vi "输出调用04.vi"(0 "输出簇":cluster{"用户名":string, "项目名称":string}, 7 "数组":string[][](array[string]), 9 "字符串":string, 11 "输出簇 2":T1) -> ()   [LabVIEW 2020]
uses:
  <vilib>/Utility/miscctls.llb/LVDateTimeRec.ctl
panel:
  out "数组 6":dbl[][](array[numeric])
  out "水质":dbl
  out "温度":dbl
  out "输出 3":dbl
  out "输出 2":dbl
  out "创建的路径":path
  out "路径 2":path
  out "路径":path
  out "错误输出":errorcluster
  out "数组 5":dbl[](array[numeric])
  out "数组 4":dbl[](array[numeric])
  out "文本":string[](array[string])
  out "数组 3":dbl[](array[numeric])
  out "数组 2":dbl[](array[numeric])
  out "错误输出 2":errorcluster caption="错误输出"
  out "元素":string
  out "数值 3":i32
  out "Numeric":i32
  in  "数值":u32
  out "输出 1":dbl
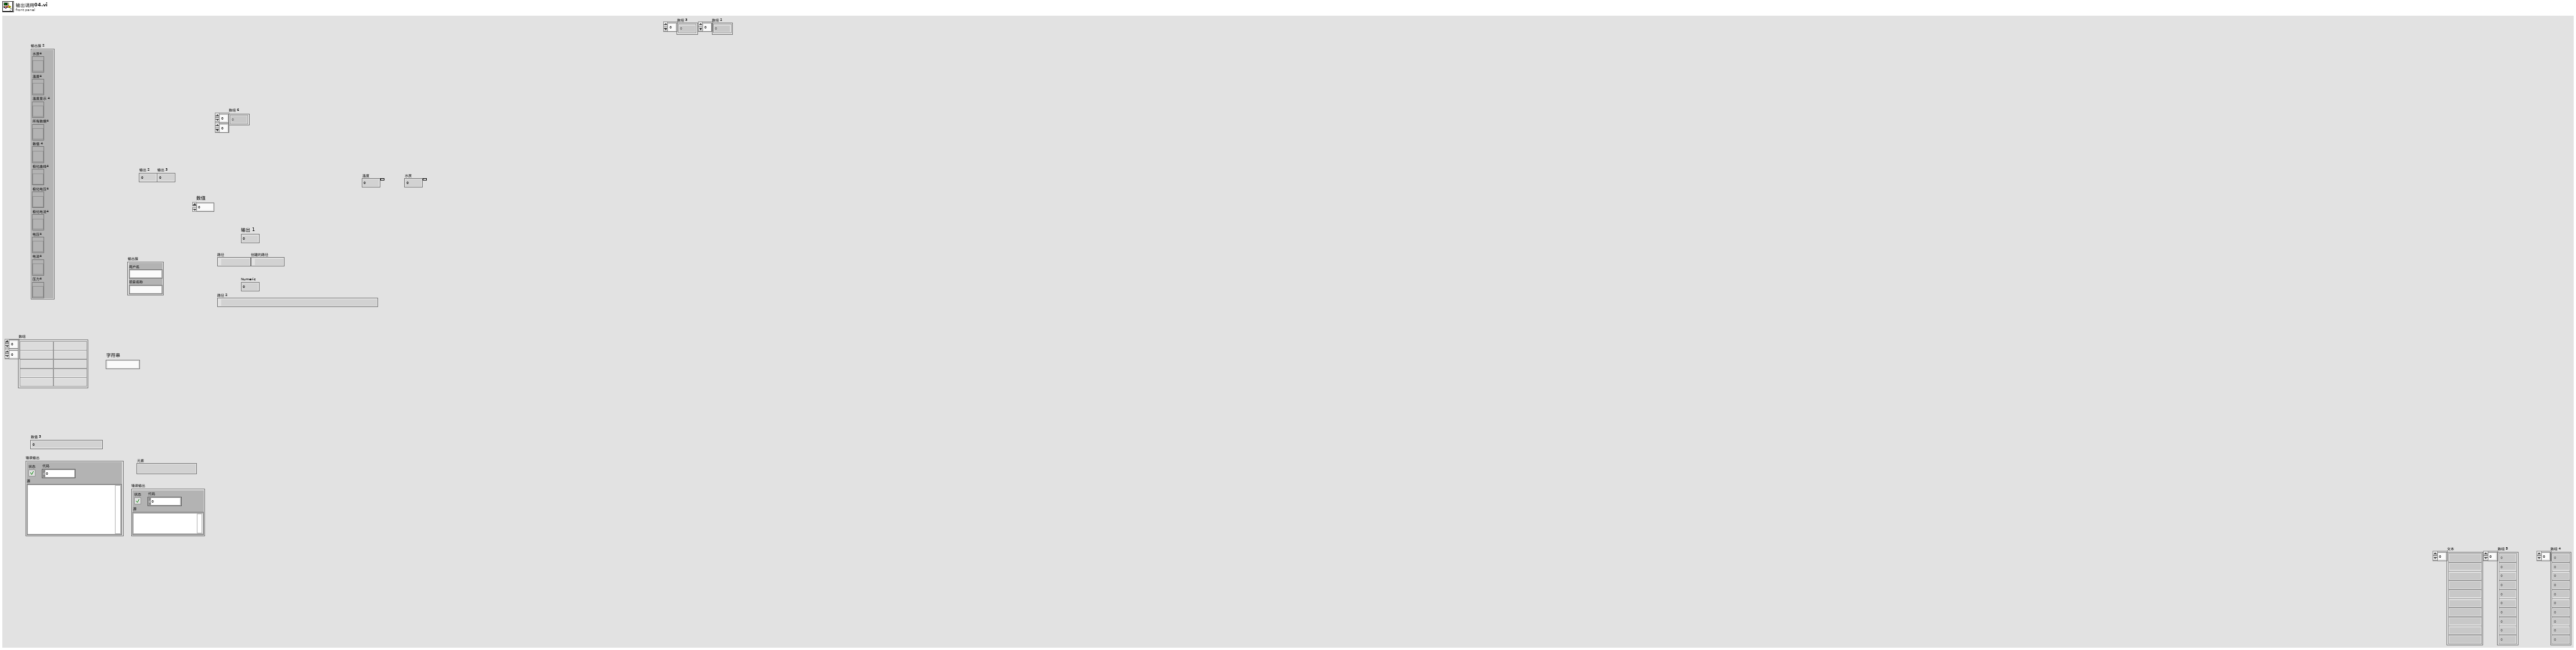
[diagram p1: front panel]
types:
  T1 = cluster{"水质4":refnum<vi>, "温度4":refnum<vi>, "温度显示 4":refnum<vi>, "所有数据4":refnum<vi>, "数值 4":refnum<vi>, "极化曲线4":refnum<vi>, "极化电压4":refnum<vi>, "极化电流4":refnum<vi>, "电压4":refnum<vi>, "电流4":refnum<vi>, "压力4":refnum<vi>}
  T2 = enum16{"open", "replace", "create", "open or create", "replace or create", "replace or create with confirmation"}
  T3 = typedef "LVDateTimeRec.ctl" = cluster{"fractional second":dbl, "second":i32, "minute":i32, "hour":i32, "day of month":i32, "month":i32, "year":i32, "day of week":i32, "day of year":i32, "DST":i32}
  T4 = enum16{"open", "open or create", "create or replace", "create", "open (read-only)"}
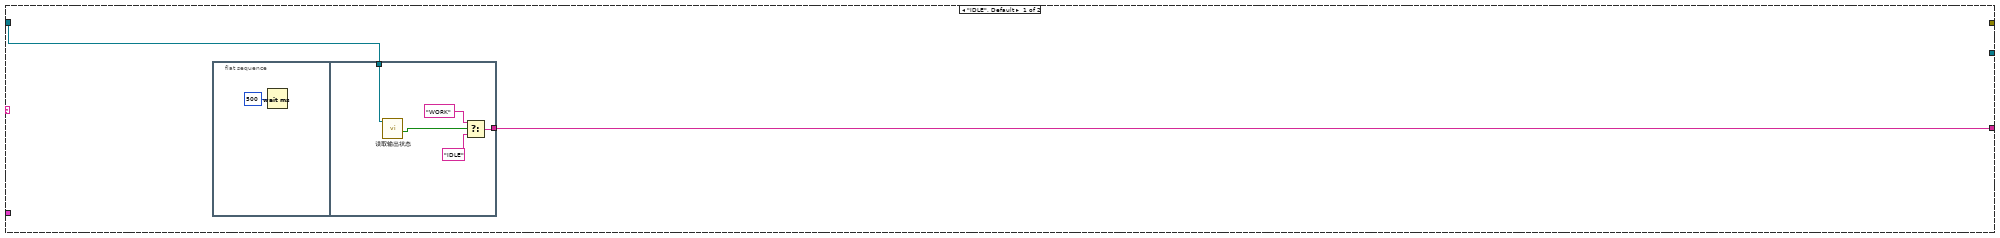
[diagram p2: hidden frame]
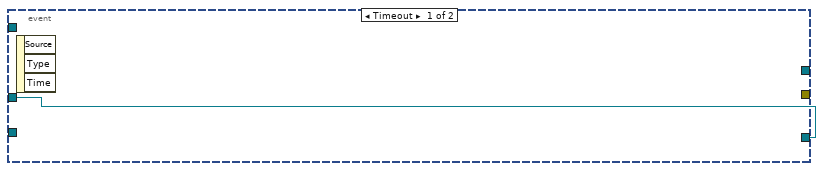
[diagram p3: hidden frame]
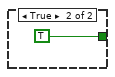
[diagram p5: hidden frame]
diagram:
  w12 = "\\" ("string")
  (unwired) dbl[] [] ("数组 4")
  n1 = Current VI's Path() -> (path=w36:path)
  n2 = Strip Path(path=w36) -> (stripped path=w35:path)  [unwired: 1 out]
  n3 = Strip Path(path=w35) -> (stripped path=w34:path)  [unwired: 1 out]
  n4 = Path To String(path=w34) -> (string=w33:string)
  n5 = Unbundle By Name("输出簇") -> ("用户名"=w9:string, "项目名称"=w8:string)
  n6 = Get Date/Time In Seconds() -> (seconds since 1Jan1904=w31:timestamp)
  n7 = Format Date/Time String(time format string (%c)="%y-%m-%d[%H-%M]", seconds (now)=w31) -> (date/time string=w11:string)  [unwired: 1 in]
  n8 = Concatenate Strings(w33, w12, "TEMPDATA\\" ("string"), w9, w12, w8, w12, w11) -> (w29:string)
  n9 = String To Path(string=w29) -> (path=w28:path)
  n10 = Create Folder(path (use dialog)=w28) -> (created path=w21:path)  [unwired: 2 in, 2 out]
  "创建的路径" <- w21
  n11 = Path To String(path=w21) -> (string=w27:string)
  n12 = Concatenate Strings(w27, "\\" ("string"), "索引.txt" ("string")) -> (w18:string)
  n13 = String To Path(string=w18) -> (path=w17:path)
  "路径 2" <- w17
  n14 = property on="输出簇 2" class="Clust (严格)"() -> ("Value"=w1:T1)  [unwired: 2 in, 2 out]
  n15 = Unbundle By Name(w1) -> ("极化曲线4"=w7:refnum<vi>)
  n16 = property on="数组 6" class="Arr (严格)"("Value"=dbl[][] [] ("数组 6")) -> (error out=w3:errorcluster)  [unwired: 2 in, 1 out]
  n17 = Open/Create/Replace File(file path (use dialog)=w17, operation (0:open)=T2."replace or create") -> (refnum out=w16:refnum<file>)  [unwired: 4 in, 2 out]
  n18 = while {
    tunnel: w45 -> [w66]
    tunnel: w16 -> [w65]
    tunnel: [w64] -> w14
    tunnel: [w63] -> w15
    shift-right: [w61] -> _
    shift-left: w7 -> [w62]
    tunnel: w3 -> [_]
    stop <- FALSE stop-if-true
    n19 = event shown="[1] \"数值\": 值改变" {
      selector: _ -> [_ _]
      dyn-events: _ -> [_ _]
      timeout: 100 -> [_ _]
      tunnel: w66 -> [_ _]
      tunnel: w65 -> [_ w84]
      tunnel: [_ w78] -> w64
      tunnel: [_ w77] -> w63
      tunnel: w62 -> [w69 w73]
      tunnel: [w69 w72] -> w61
      event Timeout {
        n20 = event-data() -> ()  [unwired: 1 in, 3 out]
      }
      event "数值": Value Change {
        n21 = event-data() -> ()  [unwired: 1 in, 6 out]
        n22 = local read "输出 3"() -> (w74:dbl)
        n23 = local read "输出 2"() -> (w75:dbl)
        n24 = property on="Numeric" class="DigNum (严格)"() -> ("Value"=w83:i32)  [unwired: 2 in, 2 out]
        n25 = Build Array(w75, w74) -> (w76:dbl[])
        n26 = Format Into String(w83) -> (resulting string=w82:string)  [unwired: 3 in, 1 out]
        n27 = property on="数组 6" class="Arr (严格)"() -> ("Value"=w71:dbl[][])  [unwired: 2 in, 2 out]
        n28 = Write to Text File(file (use dialog)=w84, text=w82) -> (refnum out=w81:refnum<file>, error out=w80:errorcluster)  [unwired: 2 in, 1 out]
        n29 = Insert Into Array(array=w71, new element=w76) -> (w70:dbl[][])  [unwired: 2 in]
        n30 = property on="数组 6" class="Arr (严格)"("Value"=w70) -> ()  [unwired: 2 in, 2 out]
        n31 = Write to Text File(file (use dialog)=w81, text="\r\n", error in=w80) -> (refnum out=w78:refnum<file>, error out=w77:errorcluster)  [unwired: 1 in, 1 out]
        n32 = property class="Arr (严格)"(reference=w73, "Value"=w70) -> (reference out=w72:refnum<vi>)  [unwired: 1 in, 1 out]
      }
    }
  }
  n33 = Close File(refnum=w14, error in=w15) -> ()  [unwired: 2 out]
  n34 = Path To String(path=w21) -> (string=w22:string)
  n35 = Concatenate Strings(w22, "\\" ("string"), "数据.txt" ("string")) -> (w20:string)
  n36 = String To Path(string=w20) -> (path=w19:path)
  "路径" <- w19
  n37 = Open/Create/Replace File(file path (use dialog)=w19, operation (0:open)=T2."replace or create" ("操作(0:open)")) -> (refnum out=w5:refnum<file>, error out=w40:errorcluster)  [unwired: 4 in, 1 out]
  n38 = flat-sequence {
    tunnel: [w89] -> w60
    tunnel: [w86] -> w57
    tunnel: w60 -> [w93]
    tunnel: [w93] -> w59
    tunnel: [w92] -> w58
    tunnel: w57 -> [w92]
    tunnel: ["字符串"] -> w43
    tunnel: w59 -> [w95]
    tunnel: w58 -> [w96]
    tunnel: [w96] -> w56
    tunnel: [w95] -> w55
    tunnel: [w94] -> w44
    tunnel: w43 -> [w94]
    tunnel: w56 -> [w103]
    tunnel: w55 -> [w104]
    tunnel: [w106] -> w54
    tunnel: [w105] -> w53
    tunnel: [w104] -> w51
    tunnel: [w103] -> w49
    tunnel: [w102] -> w45
    tunnel: w44 -> [w101]
    tunnel: w54 -> [w119]
    tunnel: w53 -> [w118]
    tunnel: [w115] -> w52
    tunnel: w51 -> [w115]
    tunnel: [w114] -> w50
    tunnel: w49 -> [w114]
    tunnel: [w109] -> w48
    tunnel: [w108] -> w47
    tunnel: ["输出簇 2"] -> w6
    tunnel: w52 -> [w148]
    tunnel: w50 -> [w152]
    tunnel: w48 -> [w151]
    tunnel: w47 -> [w150]
    tunnel: [w149] -> w46
    tunnel: [w145] -> w37
    tunnel: w6 -> [w144]
    tunnel: w46 -> [w205]
    tunnel: w37 -> [w203]
    frame #0 {
      n39 = property on="数值" class="DigNum (严格)"("Value"=i64 0 ("数值")) -> ()  [unwired: 2 in, 2 out]
      n40 = Index Array(array="数组", index (col)=5 ("禁用的索引 (列)")) -> (element=w86:string[])  [unwired: 1 in]
      n41 = Index Array(array="数组", index (col)=3 ("禁用的索引 (列)")) -> (element=w89:string[])  [unwired: 1 in]
    }
    frame #1 {
      n42 = VISA Close(VISA resource name="字符串") -> ()  [unwired: 1 in, 1 out]
    }
    frame #2 {
    }
    frame #3 {
      n43 = VISA Open(VISA resource name=w101) -> (VISA resource name=w102:refnum<visa-resource-name>, error out=w99:errorcluster)  [unwired: 4 in]
      n44 = call "remote.vi"("error in (no error)"=w99, "VISA resource name"=w102) -> ("error out"=w97:errorcluster, "VISA resource name out"=w98:refnum<visa-resource-name>)  [unwired: 8 in]
      n45 = call "enableoutput.vi"("error in (no error)"=w97, "Enable OutPut(True)"=FALSE, "VISA resource name"=w98) -> ("error out"=w105:errorcluster, "VISA resource name out"=w106:refnum<visa-resource-name>)  [unwired: 7 in]
    }
    frame #4 {
      n46 = flat-sequence {
        tunnel: w119 -> [w124]
        tunnel: w118 -> [w123]
        tunnel: [w121] -> w117
        tunnel: [w120] -> w116
        tunnel: w117 -> [w130]
        tunnel: w116 -> [w129]
        tunnel: [w126] -> w113
        tunnel: [w125] -> w112
        tunnel: w113 -> [w136]
        tunnel: w112 -> [w135]
        tunnel: [w133] -> w111
        tunnel: [w132] -> w110
        tunnel: w111 -> [w142]
        tunnel: w110 -> [w141]
        tunnel: [w138] -> w109
        tunnel: [w137] -> w108
        frame #0 {
          n47 = call "priority.vi"("error in (no error)"=w123, "字符串"="CURR", "VISA resource name"=w124) -> ("error out"=w120:errorcluster, "VISA resource name out"=w121:refnum<visa-resource-name>)  [unwired: 7 in]
        }
        frame #1 {
          n48 = call "初始化电压电流.vi"("error in (no error)"=w129, "输入 2"=0.1, "输入 1"=15.0, "VISA resource name"=w130) -> ("error out"=w125:errorcluster, "VISA resource name out"=w126:refnum<visa-resource-name>)  [unwired: 6 in]
        }
        frame #2 {
          n49 = call "限制电流.vi"("error in (no error)"=w135, "OCP Delay(0)"=3.0, "数值"=120.0 ("OCP Level(0)"), "VISA resource name"=w136) -> ("error out"=w132:errorcluster, "VISA resource name out"=w133:refnum<visa-resource-name>)  [unwired: 6 in]
        }
        frame #3 {
          n50 = call "限制电压.vi"("error in (no error)"=w141, "OVP Delay(0)"=3.0, "OVP Level(0)"=20.0, "VISA resource name"=w142) -> ("error out"=w137:errorcluster, "VISA resource name out"=w138:refnum<visa-resource-name>)  [unwired: 6 in]
        }
      }
    }
    frame #5 {
      n51 = Unbundle By Name(w144) -> ("数值 4"=w143:refnum<vi>)
      n52 = Search 1D Array(1D array=w148, element=" " ("元素")) -> (index of element=w146:i32)  [unwired: 1 in]
      n53 = for {
        N: w146 -> [_]
        tunnel: w152 -> [w174] mode=indexing
        tunnel: w148 -> [w171] mode=indexing
        tunnel: w150 -> [w169]
        shift-right: [w164] -> w149
        shift-left: w151 -> [w170]
        tunnel: [w161] -> w145
        shift-right: [w155] -> _
        shift-left: w143 -> [w156]
        i -> [w154]
        n54 = Scan From String(input string=w174) -> (output 1=w173:dbl)  [unwired: 4 in, 3 out]
        n55 = Scan From String(input string=w171) -> (output 1=w168:dbl)  [unwired: 4 in, 3 out]
        "输出 1" <- w168
        n56 = Multiply(x=w173, y=1000.0) -> (x*y=w165:dbl)
        n57 = flat-sequence {
          tunnel: w170 -> [w179]
          tunnel: w169 -> [w178]
          tunnel: w168 -> [w177]
          tunnel: [w176] -> w167
          tunnel: [w175] -> w166
          tunnel: w167 -> [w182]
          tunnel: w166 -> [w183]
          tunnel: [w181] -> w163
          tunnel: [w180] -> w162
          tunnel: w165 -> [w193]
          tunnel: w163 -> [w192]
          tunnel: [w192] -> w160
          tunnel: [w191] -> w158
          tunnel: w162 -> [w191]
          tunnel: w160 -> [w198]
          tunnel: [w198] -> w159
          tunnel: w158 -> [w197]
          tunnel: [w197] -> w157
          tunnel: w156 -> [w196]
          tunnel: [w195] -> w155
          tunnel: w153 -> [w194]
          tunnel: [w201] -> w164
          tunnel: w159 -> [w202]
          tunnel: w157 -> [w200]
          tunnel: [w199] -> w161
          frame #0 {
            n58 = call "设置电流.vi"("error in (no error)"=w178, "输入 1"=w177, "VISA resource name"=w179) -> ("error out"=w175:errorcluster, "VISA resource name out"=w176:refnum<visa-resource-name>)  [unwired: 7 in]
          }
          frame #1 {
            n59 = First Call?() -> (First Call?: T/F=w184:bool)
            n60 = case shown="真" w184 {
              tunnel: w182 -> [w185 w190]
              tunnel: w183 -> [_ w189]
              tunnel: [w185 w187] -> w181
              tunnel: [_ w186] -> w180
              frame False {
              }
              frame True {
                n61 = call "enableoutput.vi"("error in (no error)"=w189, "Enable OutPut(True)"=TRUE, "VISA resource name"=w190) -> ("error out"=w186:errorcluster, "VISA resource name out"=w187:refnum<visa-resource-name>)  [unwired: 7 in]
              }
            }
          }
          frame #2 {
            n62 = Wait (ms)(milliseconds to wait=w193) -> ()  [unwired: 1 out]
          }
          frame #3 {
            n63 = property on="数值" class="DigNum (严格)"("Val(Sgnl)"=w194) -> ()  [unwired: 2 in, 2 out]
            n64 = property class="DigNum (严格)"(reference=w196, "Val(Sgnl)"=w194) -> (reference out=w195:refnum<vi>)  [unwired: 1 in, 1 out]
          }
          frame #4 {
            n65 = call "remote.vi"("error in (no error)"=w200, "VISA resource name"=w202) -> ("error out"=w199:errorcluster, "VISA resource name out"=w201:refnum<visa-resource-name>)  [unwired: 8 in]
          }
        }
        n66 = Increment(x=w154) -> (x+1=w153:i32)
      }
    }
    frame #6 {
      n67 = flat-sequence {
        tunnel: w205 -> [w209]
        tunnel: [w208] -> w204
        tunnel: w203 -> [w206]
        tunnel: w204 -> [w210]
        frame #0 {
          n68 = call "enableoutput.vi"("error in (no error)"=w206, "Enable OutPut(True)"=FALSE, "VISA resource name"=w209) -> ("VISA resource name out"=w208:refnum<visa-resource-name>)  [unwired: 7 in, 1 out]
        }
        frame #1 {
          n69 = VISA Close(VISA resource name=w210) -> ()  [unwired: 1 in, 1 out]
        }
        frame #2 {
          n70 = flat-sequence {
            tunnel: [w227] -> w221
            tunnel: [w226] -> w220
            tunnel: [w225] -> w219
            tunnel: [w224] -> w218
            tunnel: [w223] -> w217
            tunnel: w221 -> [w270]
            tunnel: w220 -> [w269]
            tunnel: [w287] -> w211
            tunnel: [w286] -> w212
            tunnel: w219 -> [w282]
            tunnel: [w281] -> w213
            tunnel: w218 -> [w273]
            tunnel: w217 -> [w274]
            tunnel: [w271] -> w214
            tunnel: [w272] -> w215
            tunnel: [w271] -> w216
            tunnel: w216 -> [w328]
            tunnel: w215 -> [w327]
            tunnel: w214 -> [w349]
            tunnel: w213 -> [w355]
            tunnel: w212 -> [w363]
            tunnel: w211 -> [w362]
            frame #0 {
              n71 = property on="路径" class="Path"() -> ("Value"=w222:path)  [unwired: 2 in, 2 out]
              n72 = Open/Create/Replace File(file path (use dialog)=w222, operation (0:open)=T2."open" ("操作(0:open)")) -> (refnum out=w230:refnum<file>, error out=w229:errorcluster)  [unwired: 4 in, 1 out]
              n73 = while {
                tunnel: w230 -> [w266]
                tunnel: w229 -> [w264]
                tunnel: [w263] -> w228
                tunnel: [w237] -> w227 mode=indexing
                tunnel: [w236] -> w226 mode=indexing
                tunnel: [w252] -> _
                tunnel: [w240] -> w225 mode=indexing
                tunnel: [w235] -> w224 mode=indexing
                tunnel: [w234] -> w223 mode=indexing
                i -> [w233]
                stop <- w253 stop-if-true
                n74 = Read from Text File(file (use dialog)=w266, count=1 ("计数"), error in=w264) -> (refnum out=w263:refnum<file>, text=w257:string[], error out=w252:errorcluster)  [unwired: 1 in, 1 out]
                n75 = Unbundle By Name(w252) -> ("status"=w260:bool, "code"=w262:i32)
                n76 = Equal?(x=w262, y=4) -> (x = y?=w259:bool)
                n77 = Index Array(array=w257, index=0 ("索引")) -> (element=w254:string)
                "元素" <- w254
                n78 = And(x=w260, y=w259) -> (x .and. y?=w258:bool)
                n79 = case shown="假" w258 {
                  tunnel: [FALSE TRUE] -> w253
                  frame False {
                  }
                  frame True {
                  }
                }
                n80 = Search/Split String(string=w254, search string/char (-)="电流：" ("正则表达式")) -> (substring before match=w249:string, match + rest of string=w239:string)  [unwired: 1 in, 1 out]
                n81 = Scan From String(format string="%d-%d-%d %d:%d:%d" ("格式字符串"), input string=w249) -> (error out=→"错误输出 2":errorcluster, output 1=w248:i32, output 2=w247:i32, output 3=w246:i32, output 4=w245:i32, output 5=w244:i32, output 6=w243:i32)  [unwired: 8 in, 2 out]
                n82 = Bundle By Name(cluster=T3 {"fractional second"=0.9035696983337402, "second"=34, "minute"=35, "hour"=15, "day of month"=21, "month"=2, "year"=2022, "day of week"=2, "day of year"=52, "DST"=0} ("日期时间记录"), "second"=w243, "minute"=w244, "hour"=w245, "day of month"=w246, "month"=w247, "year"=w248) -> (w241:T3)
                n83 = Scan From String(format string="电流：%f 电压：%f 温度：%f 水质：%f" ("格式字符串"), input string=w239) -> (error out=w232:errorcluster, output 1=w237:dbl, output 2=w236:dbl, output 3=w235:dbl, output 4=w234:dbl)  [unwired: 6 in, 2 out]
                n84 = call <vilib>:"Clear Errors.vi"("error in (no error)"=w232) -> ()  [unwired: 5 in, 2 out]
                n85 = Date/Time To Seconds(2:w241) -> (0:w240:timestamp)  [unwired: 1 in]
                "数值 3" <- w233
              }
              n86 = Close File(refnum=w228) -> ()  [unwired: 1 in, 2 out]
            }
            frame #1 {
              n87 = Array Size(array=w269) -> (size(s)=w289:i32)
              n88 = Array Size(array=w270) -> (size(s)=w292:i32)
              n89 = Array Size(array=w282) -> (size(s)=w284:i32)
              n90 = Decrement(x=w289) -> (x-1=w290:i32)
              n91 = Decrement(x=w292) -> (x-1=w291:i32)
              n92 = Decrement(x=w284) -> (x-1=w285:i32)
              n93 = Array Size(array=w273) -> (size(s)=w280:i32)
              n94 = Array Size(array=w274) -> (size(s)=w279:i32)
              n95 = Decrement(x=w280) -> (x-1=w278:i32)
              n96 = Decrement(x=w279) -> (x-1=w275:i32)
              n97 = Delete From Array(array=w273, length=1 ("长度"), index=w278) -> (array with subset deleted=w271:dbl[])  [unwired: 1 out]
              n98 = Delete From Array(array=w269, length=1 ("长度"), index=w290) -> (array with subset deleted=w286:dbl[])  [unwired: 1 out]
              n99 = Delete From Array(array=w270, length=1 ("长度"), index=w291) -> (array with subset deleted=w287:dbl[])  [unwired: 1 out]
              n100 = Delete From Array(array=w282, length=1 ("长度"), index=w285) -> (array with subset deleted=w281:timestamp[])  [unwired: 1 out]
              n101 = Delete From Array(array=w274, length=1 ("长度"), index=w275) -> (array with subset deleted=w272:dbl[])  [unwired: 1 out]
              "数组 3" <- w270
              "数组 2" <- w269
            }
            frame #2 {
              w314 = "极化" ("组名称输入（无标题）")
              w340 = "数据" ("组名称")
              n102 = property on="创建的路径" class="Path"() -> ("Value"=w294:path)  [unwired: 2 in, 2 out]
              n103 = Array Max & Min(array=w349) -> (max value=w321:dbl, max index (indices)=w319:i32, min value=w320:dbl, min index (indices)=w318:i32)
              n104 = Array Max & Min(array=w327) -> (max value=w325:dbl, max index (indices)=w323:i32, min value=w324:dbl, min index (indices)=w322:i32)
              n105 = Array Size(array=w355) -> (size(s)=w354:i32)
              n106 = Array Max & Min(array=w363) -> (max value=w376:dbl, max index (indices)=w371:i32, min value=w375:dbl, min index (indices)=w370:i32)
              n107 = Array Max & Min(array=w362) -> (max value=w378:dbl, max index (indices)=w372:i32, min value=w379:dbl, min index (indices)=w373:i32)
              n108 = Index Array(array=w355, index=0 ("索引")) -> (element=w352:timestamp)
              n109 = Build Array(w325, w324, w323, w322) -> (w336:dbl[])
              n110 = Build Array(w321, w320, w319, w318) -> (w337:dbl[])
              n111 = Decrement(x=w354) -> (x-1=w353:i32)
              n112 = Build Array(w375, w376, w371, w370) -> (w374:dbl[])
              n113 = Build Array(w379, w378, w373, w372) -> (w377:dbl[])
              n114 = Path To String(path=w294) -> (string=w295:string)
              n115 = Index Array(array=w355, index=w353) -> (element=w351:timestamp)
              n116 = Get Date/Time In Seconds() -> (seconds since 1Jan1904=w395:timestamp)
              n117 = Format Date/Time String(time format string (%c)="%Y-%m-%d-%H-%M-%S" ("时间格式字符串(%c)"), seconds (now)=w395) -> (date/time string=w297:string)  [unwired: 1 in]
              n118 = Concatenate Strings(w295, "\\" ("字符串"), w297, ".tdms" ("字符串")) -> (w396:string)
              n119 = String To Path(string=w396) -> (path=w397:path)
              n120 = Build Array(w352, w351) -> (w350:timestamp[])
              n121 = TDMS Open(5:FALSE ("创建索引文件？(T)"), 10:T4."create or replace" ("操作(0:open)"), 11:w397) -> (0:w303:errorcluster, 3:w305:refnum<k34>)  [unwired: 4 in]
              n122 = Build Array("电解水实验" ("组名称"), "孙成，王彪" ("组名称"), w297, "极化曲线" ("组名称")) -> (w296:string[])
              n123 = TDMS Set Properties(5:w296, 7:string[] ["Title", "Author", "Date/Time", "type"] ("属性名称"), 8:w303, 11:w305) -> (0:w302:errorcluster, 3:w304:refnum<k34>)  [unwired: 2 in, 2 out]
              n124 = TDMS Set Properties(5:w350, 7:string[] ["最小值", "最大值"] ("属性名称"), 8:w302, 9:"测试时间" ("通道名称"), 10:w340, 11:w304) -> (0:w386:errorcluster, 3:w387:refnum<k34>)  [unwired: 2 out]
              n125 = TDMS Set Properties(5:w377, 7:string[] ["最小值", "最大值", "最小索引", "最大索引"] ("属性名称"), 8:w386, 9:"电流" ("通道名称"), 10:w340, 11:w387) -> (0:w380:errorcluster, 3:w383:refnum<k34>)  [unwired: 2 out]
              n126 = TDMS Set Properties(5:w374, 7:string[] ["最小值", "最大值", "最小索引", "最大索引"] ("属性名称"), 8:w380, 9:"电压" ("通道名称"), 10:w340, 11:w383) -> (0:w343:errorcluster, 3:w344:refnum<k34>)  [unwired: 2 out]
              n127 = TDMS Set Properties(5:w337, 7:string[] ["最小值", "最大值", "最小索引", "最大索引"] ("属性名称"), 8:w343, 9:"温度" ("通道名称"), 10:w340, 11:w344) -> (0:w341:errorcluster, 3:w342:refnum<k34>)  [unwired: 2 out]
              n128 = TDMS Set Properties(5:w336, 7:string[] ["最小值", "最大值", "最小索引", "最大索引"] ("属性名称"), 8:w341, 9:"水质" ("通道名称"), 10:w340, 11:w342) -> (0:w338:errorcluster, 3:w339:refnum<k34>)  [unwired: 2 out]
              n129 = TDMS Write(0:w339, 5:"数据" ("组名称输入（无标题）"), 7:string[] ["电流"] ("通道名输入（无标题）"), 9:w362, 11:w338) -> (4:w366:refnum<k34>, 15:w365:errorcluster)  [unwired: 1 in, 2 out]
              n130 = TDMS Write(0:w366, 5:"数据" ("组名称输入（无标题）"), 7:string[] ["电压"] ("通道名输入（无标题）"), 9:w363, 11:w365) -> (4:w358:refnum<k34>, 15:w357:errorcluster)  [unwired: 1 in, 2 out]
              n131 = TDMS Write(0:w358, 5:"数据" ("组名称输入（无标题）"), 7:string[] ["测试时间"] ("通道名输入（无标题）"), 9:w355, 11:w357) -> (4:w330:refnum<k34>, 15:w329:errorcluster)  [unwired: 1 in, 2 out]
              n132 = TDMS Write(0:w330, 5:"数据" ("组名称输入（无标题）"), 7:string[] ["温度"] ("通道名输入（无标题）"), 9:w328, 11:w329) -> (4:w326:refnum<k34>, 15:w335:errorcluster)  [unwired: 1 in, 2 out]
              n133 = TDMS Write(0:w326, 5:"数据" ("组名称输入（无标题）"), 7:string[] ["水质"] ("通道名输入（无标题）"), 9:w327, 11:w335) -> (4:w311:refnum<k34>, 15:w310:errorcluster)  [unwired: 1 in, 2 out]
              n134 = flat-sequence {
                tunnel: [w399] -> w317
                tunnel: w317 -> [w406]
                tunnel: [w405] -> w307
                tunnel: [w404] -> w306
                frame #0 {
                  n135 = property on="路径 2" class="Path"() -> ("Value"=w398:path)  [unwired: 2 in, 2 out]
                  n136 = Open/Create/Replace File(file path (use dialog)=w398, operation (0:open)=T2."open" ("操作(0:open)")) -> (refnum out=w403:refnum<file>)  [unwired: 4 in, 2 out]
                  n137 = Read from Text File(file (use dialog)=w403, count=-1 ("计数")) -> (refnum out=w400:refnum<file>, text=w399:string[])  [unwired: 2 in, 2 out]
                  "文本" <- w399
                  n138 = Close File(refnum=w400) -> ()  [unwired: 1 in, 2 out]
                }
                frame #1 {
                  n139 = for {
                    tunnel: w406 -> [w415] mode=indexing
                    tunnel: [w413] -> w405 mode=indexing
                    tunnel: [w412] -> w404 mode=indexing
                    n140 = Scan From String(format string="%d" ("格式字符串"), input string=w415) -> (output 1=w411:i32)  [unwired: 3 in, 3 out]
                    n141 = property on="数组 3" class="Arr (严格)"() -> ("Value"=w407:dbl[])  [unwired: 2 in, 2 out]
                    n142 = Decrement(x=w411) -> (x-1=w410:i32)
                    n143 = Decrement(x=w411) -> (x-1=w409:i32)
                    n144 = Index Array(array=w407, index=w410) -> (element=w413:dbl)
                    n145 = property on="数组 2" class="Arr (严格)"() -> ("Value"=w408:dbl[])  [unwired: 2 in, 2 out]
                    n146 = Index Array(array=w408, index=w409) -> (element=w412:dbl)
                  }
                  "数组 5" <- w405
                  "数组 4" <- w404
                }
              }
              n147 = TDMS Write(0:w311, 5:w314, 7:string[] ["电流"] ("通道名输入（无标题）"), 9:w307, 11:w310) -> (4:w316:refnum<k34>, 15:w315:errorcluster)  [unwired: 1 in, 2 out]
              n148 = TDMS Write(0:w316, 5:w314, 7:string[] ["电压"] ("通道名输入（无标题）"), 9:w306, 11:w315) -> (4:w309:refnum<k34>, 15:w308:errorcluster)  [unwired: 1 in, 2 out]
              n149 = TDMS Close(8:w308, 11:w309) -> (0:→"错误输出":errorcluster)  [unwired: 1 out]
            }
          }
        }
        frame #3 {
          n150 = Request Deallocation(TRUE ("标志")) -> ()
        }
        frame #4 {
          n151 = Stop(stop? (T)=TRUE ("停止？(T)")) -> ()
        }
      }
    }
  }
  n152 = property on="输出簇 2" class="Clust (严格)"() -> ("Value"=w2:T1)  [unwired: 2 in, 2 out]
  n153 = while {
    shift-right: [w421] -> _
    shift-left: "IDLE" -> [w427]
    tunnel: w45 -> [w426]
    tunnel: w5 -> [w425]
    tunnel: w40 -> [w424]
    tunnel: [w423] -> w39
    tunnel: [w422] -> w38
    tunnel: w2 -> [w418]
    i -> [w420]
    stop <- FALSE stop-if-true
    n154 = Wait (ms)(milliseconds to wait=u32 500 ("等待时间（毫秒）")) -> ()  [unwired: 1 out]
    n155 = case shown="\"WORK\"" w427 {
      tunnel: [w430 w481] -> w421
      tunnel: w426 -> [w429 w489]
      tunnel: w425 -> [_ w488]
      tunnel: w424 -> [_ w486]
      tunnel: [_ w483] -> w423
      tunnel: [_ w482] -> w422
      tunnel: w418 -> [_ w466]
      frame "IDLE", Default {
        n156 = flat-sequence {
          tunnel: [w433] -> w430
          tunnel: w429 -> [w432]
          frame #0 {
            n157 = Wait (ms)(milliseconds to wait=u32 500 ("等待时间（毫秒）")) -> ()  [unwired: 1 out]
          }
          frame #1 {
            n158 = call "读取输出状态.vi"("VISA resource name"=w432) -> ("x = y?"=w436:bool)  [unwired: 7 in, 3 out]
            n159 = Select(t="WORK", s=w436, f="IDLE") -> (s? t:f=w433:string)
          }
        }
      }
      frame "WORK" {
        n160 = Unbundle By Name(w466) -> ("所有数据4"=w444:refnum<vi>, "极化电压4"=w442:refnum<vi>, "极化电流4"=w465:refnum<vi>, "电压4"=w464:refnum<vi>, "电流4"=w463:refnum<vi>, "水质4"=w443:refnum<vi>, "温度4"=w441:refnum<vi>)  [unwired: 3 out]
        n161 = flat-sequence {
          tunnel: [w499] -> w492
          tunnel: [w498] -> w491
          tunnel: w489 -> [w497]
          tunnel: w488 -> [w495]
          tunnel: [w496] -> w487
          tunnel: w486 -> [w496]
          tunnel: [w495] -> w485
          tunnel: [w493] -> w484
          tunnel: w465 -> [w494]
          tunnel: [w493] -> w459
          tunnel: w492 -> [w511]
          tunnel: w491 -> [w510]
          tunnel: [w502] -> w480
          tunnel: [w508] -> w478
          tunnel: [w507] -> w476
          tunnel: w487 -> [w505]
          tunnel: w485 -> [w506]
          tunnel: [w506] -> w474
          tunnel: [w505] -> w472
          tunnel: [w504] -> w470
          tunnel: w484 -> [w504]
          tunnel: [w502] -> w468
          tunnel: [w502] -> w462
          tunnel: [w503] -> w460
          tunnel: w459 -> [w503]
          tunnel: [w502] -> w457
          tunnel: w442 -> [w501]
          tunnel: w480 -> [w529]
          tunnel: [w529] -> w479
          tunnel: w478 -> [w528]
          tunnel: [w528] -> w477
          tunnel: w476 -> [w527]
          tunnel: [w527] -> w475
          tunnel: w474 -> [w526]
          tunnel: [w526] -> w473
          tunnel: w472 -> [w525]
          tunnel: [w525] -> w471
          tunnel: w470 -> [w524]
          tunnel: [w524] -> w469
          tunnel: w468 -> [w523]
          tunnel: [w523] -> w467
          tunnel: w464 -> [w522]
          tunnel: w463 -> [w514]
          tunnel: w462 -> [w519]
          tunnel: [w513] -> w461
          tunnel: w460 -> [w513]
          tunnel: [w512] -> w458
          tunnel: w457 -> [w512]
          tunnel: w479 -> [_]
          tunnel: [w597] -> w456
          tunnel: w477 -> [w597]
          tunnel: w475 -> [w580]
          tunnel: w473 -> [w584]
          tunnel: w471 -> [w583]
          tunnel: w469 -> [w582]
          tunnel: w467 -> [w568]
          tunnel: [w581] -> w454
          tunnel: [w580] -> w452
          tunnel: [w579] -> w482
          tunnel: [w564] -> w450
          tunnel: w461 -> [w564]
          tunnel: [w563] -> w448
          tunnel: w458 -> [w563]
          tunnel: [w556] -> w446
          tunnel: w443 -> [w555]
          tunnel: w441 -> [w536]
          tunnel: [w533] -> w439
          tunnel: [w532] -> w437
          tunnel: w456 -> [w605]
          tunnel: [w605] -> w455
          tunnel: w454 -> [w604]
          tunnel: [w604] -> w453
          tunnel: w452 -> [w603]
          tunnel: [w603] -> w451
          tunnel: w450 -> [w602]
          tunnel: [w602] -> w449
          tunnel: w448 -> [w601]
          tunnel: [w601] -> w447
          tunnel: w446 -> [w600]
          tunnel: [w600] -> w445
          tunnel: [w599] -> w440
          tunnel: w439 -> [w599]
          tunnel: [w598] -> w438
          tunnel: w437 -> [w598]
          tunnel: [w626] -> w490
          tunnel: w455 -> [w626]
          tunnel: w453 -> [w625]
          tunnel: w451 -> [w624]
          tunnel: [w623] -> w483
          tunnel: w449 -> [w618]
          tunnel: w447 -> [w615]
          tunnel: w445 -> [w609]
          tunnel: w444 -> [w608]
          tunnel: w440 -> [w607]
          tunnel: w438 -> [w606]
          tunnel: w490 -> [w631]
          tunnel: [w627] -> w481
          frame #0 {
            w500 = 0 items=["Current", "Power", "Voltage", "Capacity", "Temperature", "Time"] ("Fetch Type")
            n162 = call "fetch.vi"("Fetch Type"=w500, "VISA resource name"=w497) -> ("error out"=w498:errorcluster, "输出 1"=w493:dbl, "VISA resource name out"=w499:refnum<visa-resource-name>)  [unwired: 7 in]
            "输出 2" <- w493
            n163 = property class="DigNum (严格)"(reference=w494, "Value"=w493) -> ()  [unwired: 1 in, 2 out]
          }
          frame #1 {
            w509 = 2 items=["Current", "Power", "Voltage", "Capacity", "Temperature", "Time"] ("Fetch Type")
            n164 = call "fetch.vi"("error in (no error)"=w510, "Fetch Type"=w509, "VISA resource name"=w511) -> ("error out"=w507:errorcluster, "输出 1"=w502:dbl, "VISA resource name out"=w508:refnum<visa-resource-name>)  [unwired: 6 in]
            "输出 3" <- w502
            n165 = property class="DigNum (严格)"(reference=w501, "Value"=w502) -> ()  [unwired: 1 in, 2 out]
          }
          frame #2 {
            n166 = property class="Arr (严格)"(reference=w522) -> (reference out=w521:refnum<vi>, "Value"=w520:dbl[])  [unwired: 1 in, 1 out]
            n167 = Insert Into Array(array=w520, new element=w519) -> (w518:dbl[])  [unwired: 1 in]
            n168 = property class="Arr (严格)"(reference=w514) -> (reference out=w515:refnum<vi>, "Value"=w516:dbl[])  [unwired: 1 in, 1 out]
            n169 = property class="Arr (严格)"(reference=w521, "Value"=w518) -> ()  [unwired: 1 in, 2 out]
            n170 = Insert Into Array(array=w516, new element=w513) -> (w517:dbl[])  [unwired: 1 in]
            n171 = property class="Arr (严格)"(reference=w515, "Value"=w517) -> ()  [unwired: 1 in, 2 out]
          }
          frame #3 {
            (unwired) "时间：" ("字符串")
            n172 = Get Date/Time String() -> (date string=w542:string, time string=w540:string)  [unwired: 3 in]
            n173 = Get Date/Time String() -> (date string=w560:string, time string=w562:string)  [unwired: 3 in]
            n174 = call <vilib>:"Space Constant.vi"() -> ("String"=w554:string)
            n175 = Get Date/Time In Seconds() -> (seconds since 1Jan1904=w596:timestamp)
            n176 = Format Into String(w582) -> (resulting string=w593:string)  [unwired: 3 in, 1 out]
            n177 = Concatenate Strings(w542, "  " ("字符串"), w540) -> (w546:string)
            n178 = Concatenate Strings(w554, "电流：" ("字符串"), w593) -> (w592:string)
            n179 = Concatenate Strings(w560, "  " ("字符串"), w562) -> (w556:string)
            n180 = Format Date/Time String(time format string (%c)="%Y-%m-%d %H:%M:%S" ("时间格式字符串(%c)"), seconds (now)=w596) -> (date/time string=w594:string)  [unwired: 1 in]
            n181 = Write to Text File(file (use dialog)=w584, text=w594, error in=w583) -> (refnum out=w591:refnum<file>, error out=w590:errorcluster)  [unwired: 1 in, 1 out]
            n182 = Write to Text File(file (use dialog)=w591, text=w592, error in=w590) -> (refnum out=w587:refnum<file>, error out=w586:errorcluster)  [unwired: 1 in, 1 out]
            n183 = call <vilib>:"Space Constant.vi"() -> ("String"=w553:string)
            n184 = Format Into String(w568) -> (resulting string=w588:string)  [unwired: 3 in, 1 out]
            n185 = property on="温度" class="DigNum (严格)"() -> ("Value"=w534:dbl)  [unwired: 2 in, 2 out]
            n186 = Format Into String(format string="%.2f" ("格式字符串"), w534) -> (resulting string=w532:string)  [unwired: 2 in, 1 out]
            n187 = Concatenate Strings(w532, "°C" ("字符串")) -> (w544:string)
            n188 = property class="Arr (严格)"(reference=w536) -> (reference out=w537:refnum<vi>, "Value"=w539:string[][])  [unwired: 1 in, 1 out]
            n189 = property class="Arr (严格)"(reference=w555) -> (reference out=w567:refnum<vi>, "Value"=w565:string[][])  [unwired: 1 in, 1 out]
            n190 = Concatenate Strings(w553, "电压：" ("字符串"), w588) -> (w589:string)
            n191 = Write to Text File(file (use dialog)=w587, text=w589, error in=w586) -> (refnum out=w574:refnum<file>, error out=w573:errorcluster)  [unwired: 1 in, 1 out]
            n192 = Build Array(w546, w544) -> (w545:string[])
            n193 = call <vilib>:"Space Constant.vi"() -> ("String"=w552:string)
            n194 = Format Into String(w534) -> (resulting string=w578:string)  [unwired: 3 in, 1 out]
            n195 = property on="水质" class="DigNum (严格)"() -> ("Value"=w535:dbl)  [unwired: 2 in, 2 out]
            n196 = Format Into String(format string="%.2f" ("格式字符串"), w535) -> (resulting string=w533:string)  [unwired: 2 in, 1 out]
            n197 = Concatenate Strings(w533, "MΩ*cm" ("字符串")) -> (w558:string)
            n198 = Build Array(w556, w558) -> (w557:string[])
            n199 = Insert Into Array(array=w539, new element=w545) -> (w538:string[][])  [unwired: 2 in]
            n200 = Insert Into Array(array=w565, new element=w557) -> (w566:string[][])  [unwired: 2 in]
            n201 = Concatenate Strings(w552, "温度：" ("字符串"), w578) -> (w577:string)
            n202 = Write to Text File(file (use dialog)=w574, text=w577, error in=w573) -> (refnum out=w572:refnum<file>, error out=w571:errorcluster)  [unwired: 1 in, 1 out]
            n203 = call <vilib>:"Space Constant.vi"() -> ("String"=w551:string)
            n204 = Format Into String(w535) -> (resulting string=w575:string)  [unwired: 3 in, 1 out]
            n205 = property class="Arr (严格)"(reference=w537, "Value"=w538) -> ()  [unwired: 1 in, 2 out]
            n206 = property class="Arr (严格)"(reference=w567, "Value"=w566) -> ()  [unwired: 1 in, 2 out]
            n207 = Concatenate Strings(w551, "水质：" ("字符串"), w575) -> (w576:string)
            n208 = Write to Text File(file (use dialog)=w572, text=w576, error in=w571) -> (refnum out=w570:refnum<file>, error out=w569:errorcluster)  [unwired: 1 in, 1 out]
            n209 = Write to Text File(file (use dialog)=w570, text="\r\n", error in=w569) -> (refnum out=w579:refnum<file>, error out=w581:errorcluster)  [unwired: 1 in, 1 out]
          }
          frame #4 {
          }
          frame #5 {
            n210 = Merge Errors(w624, w625) -> (w623:errorcluster)
            n211 = Multiply(x=w615, y=w618) -> (x*y=w612:dbl)
            n212 = Format Into String(format string="%.2f" ("格式字符串"), w618) -> (resulting string=w617:string)  [unwired: 2 in, 1 out]
            n213 = property class="Arr (严格)"(reference=w608) -> (reference out=w621:refnum<vi>, "Value"=w622:string[][])  [unwired: 1 in, 1 out]
            n214 = Format Into String(format string="%.2f" ("格式字符串"), w615) -> (resulting string=w614:string)  [unwired: 2 in, 1 out]
            n215 = Format Into String(format string="%.2f" ("格式字符串"), w612) -> (resulting string=w611:string)  [unwired: 2 in, 1 out]
            n216 = Build Array(w609, w617, w614, w611, w606, w607) -> (w610:string[])
            n217 = Insert Into Array(array=w622, new element=w610) -> (w620:string[][])  [unwired: 2 in]
            n218 = property class="Arr (严格)"(reference=w621, "Value"=w620) -> ()  [unwired: 1 in, 2 out]
          }
          frame #6 {
            n219 = call "读取输出状态.vi"("VISA resource name"=w631) -> ("x = y?"=w630:bool)  [unwired: 7 in, 3 out]
            n220 = Select(t="WORK", s=w630, f="IDLE") -> (s? t:f=w627:string)
          }
        }
      }
    }
    "Numeric" <- w420
  }
  n221 = Close File(refnum=w38, error in=w39) -> ()  [unwired: 2 out]
